vi "DRT.vi"(0 "System no.":i32=1 min=1 max=4 step=1, 2 "DataRecorderTable":i32[](array[numeric]), 5 "error in":errorcluster, 6 "Trigger source":i32[](array[numeric]), 10 "Value":string[](array[string])) -> (14 "Controller error":bool, 19 "error out":errorcluster)   [LabVIEW 2020]
doc: "This VI defines a trigger source for data recorder tables, waits 100 ms and queries ERR?. See GCS DLL manual or User manual for available trigger sources and values. Controller error is TRUE if selected system reports error code not equal to 0. \n\nC-866: See C-866_GCS_Commands_SM150E.pdf for available trigger sources and values. DataRecorderTable = 0 (the specified trigger source is set for all data recorder tables).\n\nC-413, C-843, C-867, C-877, C-884, C-891, E-518, E-709, E-712, E-754, E-861, E-871, E-873, E-874, Mercury_GCS: See user manual for available trigger sources and values. DataRecorderTable = 0 (the specified trigger source is set for all data recorder tables).\n\nE-712, E-725, E-753: See user manual for available trigger sources and values. The specified trigger source is set for all data recorder tables. \n\nE-727, E-754: See user manual for available trigger sources and values. The specified trigger source is set for all data recorder tables. \n\nC-887, F-206, M-8X0: Only for GCS syntax version = GCS 2.0 or higher (check with CSV?.vi. If CSV?.vi is not supported, syntax version is GCS 1.0). See user manual for available trigger sources and values. DataRecorderTable = 0 (the specified trigger source is set for all data recorder tables)."
panel:
  # "This vi defines a trigger source for data recorder tables, waits 100 ms and queries ERR?. \nSee GCS DLL manual or User manual  for available trigger sources and values. Controller \nerror is TRUE if selected system reports error code not equal to 0."
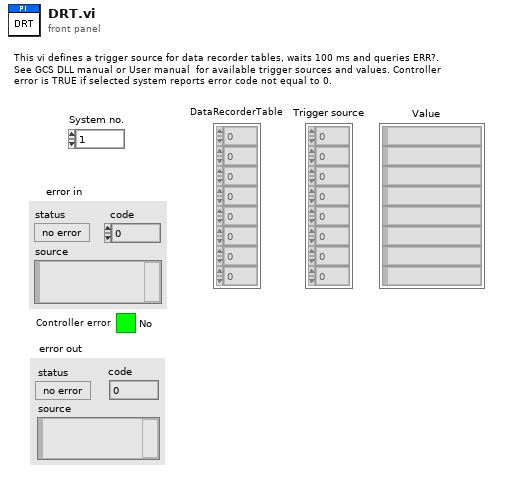
[diagram p1: front panel]
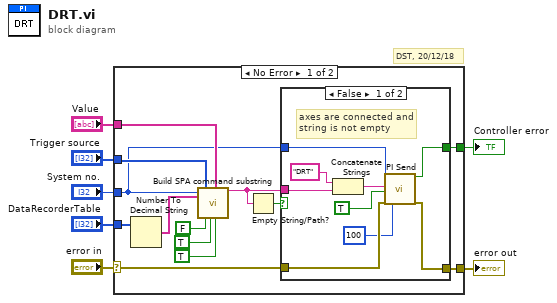
[diagram p0: block diagram]
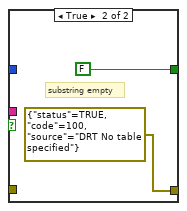
[diagram p2: hidden frame]
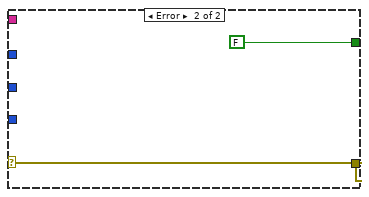
[diagram p3: hidden frame]
diagram:
  # "DST, 20/12/18"
  n1 = case shown="No Error" "error in" {
    selector: "error in" -> [w11 w33]
    tunnel: [w20 w33] -> w7
    tunnel: "System no." -> [w17 _]
    tunnel: "DataRecorderTable" -> [w16 _]
    tunnel: "Trigger source" -> [w19 _]
    tunnel: "Value" -> [w18 _]
    tunnel: [w10 FALSE ("Controller error")] -> w1
    frame No Error {
      n2 = Number To Decimal String(number=w16) -> (decimal integer string=w15:string[])  [unwired: 1 out]
      n3 = call "Build SPA command substring.vi"("System no."=w17, "Axes to set"=w15, "Parameter number"=w19, "Parameter no. format \n(Decimal: FALSE)"=FALSE ("Parameter no. format \n(Decimal: FALSE)"), "Parameter format \n(Num.: FALSE)"=TRUE ("Parameter format \n(Num.: FALSE)"), "Parameter strings"=w18, "With space?"=TRUE) -> ("SPA command substring"=w9:string)  [unwired: 3 in, 9 out]
      n4 = Empty String/Path?(string/path=w9) -> (empty?=w8:bool)
      n5 = case shown="False" w8 {
        tunnel: w9 -> [w28 _]
        tunnel: [w21 errorcluster {"status"=TRUE, "code"=100, "source"="DRT No table specified"} ("error out")] -> w20
        tunnel: w11 -> [w25 _]
        tunnel: w17 -> [w24 _]
        tunnel: [w22 FALSE ("Controller error")] -> w10
        frame False {
          # "axes are connected and\nstring is not empty"
          n6 = Concatenate Strings("DRT", w28) -> (w26:string)
          n7 = call "PI Send.vi"("System no."=w24, "String to send"=w26, "Attach termination char.?"=TRUE ("Attach Linefeed?"), "error in"=w25, "Delay before error check (ms)"=u32 100 ("milliseconds to wait")) -> ("Controller error"=w22:bool, "error out"=w21:errorcluster)  [unwired: 1 in, 12 out]
        }
        frame True {
          # "substring empty"
        }
      }
    }
    frame Error {
    }
  }
  "error out" <- w7
  "Controller error" <- w1
